vi "identColor.vi"(7 "Parâmetros Ini":T2={"Gyro Port"=0, "Sensor - Left"=3, "Sensor - Right"=2, "     Color \nSensor Port"=1, "Kp Front"=0.5, "Motor speed"=-15, "Distance to street"=0.0, "Motor speed turns"=16, "Kp Curvas"=0.0} {"Kp Front" format="%.3f"; "Color \nSensor Port" items=["Port 1", "Port 2", "Port 3", "Port 4"]; "Sensor - Right" items=["Port 1", "Port 2", "Port 3", "Port 4"]; "Sensor - Left" items=["Port 1", "Port 2", "Port 3", "Port 4"]; "Gyro Port" items=["Port 1", "Port 2", "Port 3", "Port 4"]}, 11 "NXT/EV3":T1) -> (1 "Collor":T4)   [LabVIEW 2016]
uses:
  <vilib>/NXT/Subs/LVHSConnector.ctl
  <vilib>/NXT/LegoClasses/BrickReference/BrickReference.lvclass
  <vilib>/NXT/Subs/ColorSensorColors.ctl
  parametros.ctl
  <vilib>/NXT/Block Support/NXT_InputPort.ctl
panel:
  out "NXT/EV3 2":T1
  out "Detected Color":T4
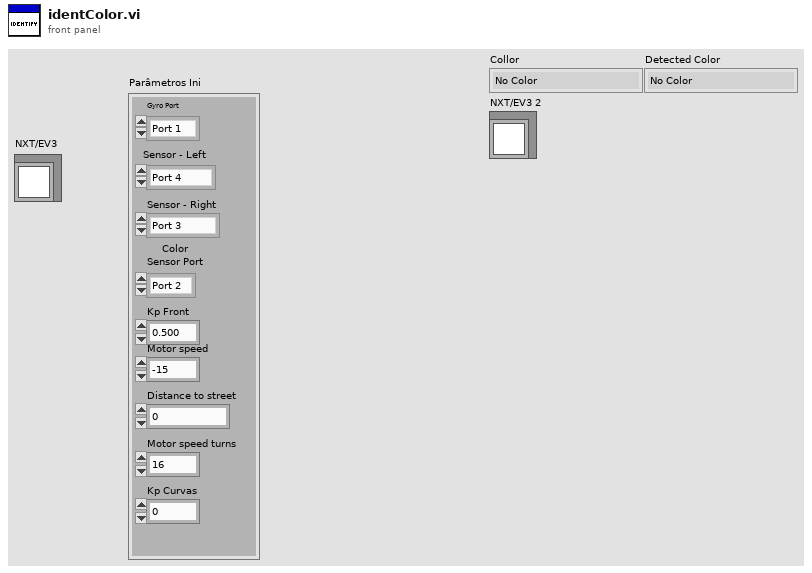
[diagram p1: front panel]
types:
  T1 = typedef "LVHSConnector.ctl" = refnum<class "BrickReference.lvclass">
  T2 = typedef "parametros.ctl" = cluster{"Gyro Port":T3, "Sensor - Left":T3, "Sensor - Right":T3, "     Color \nSensor Port":T3, "Kp Front":dbl, "Motor speed":i32, "Distance to street":dbl, "Motor speed turns":i32, "Kp Curvas":dbl}
  T3 = typedef "NXT_InputPort.ctl" = u32
  T4 = typedef "ColorSensorColors.ctl" = enum16{"No Color", "Black", "Blue", "Green", "Yellow", "Red", "White", "Brown"}
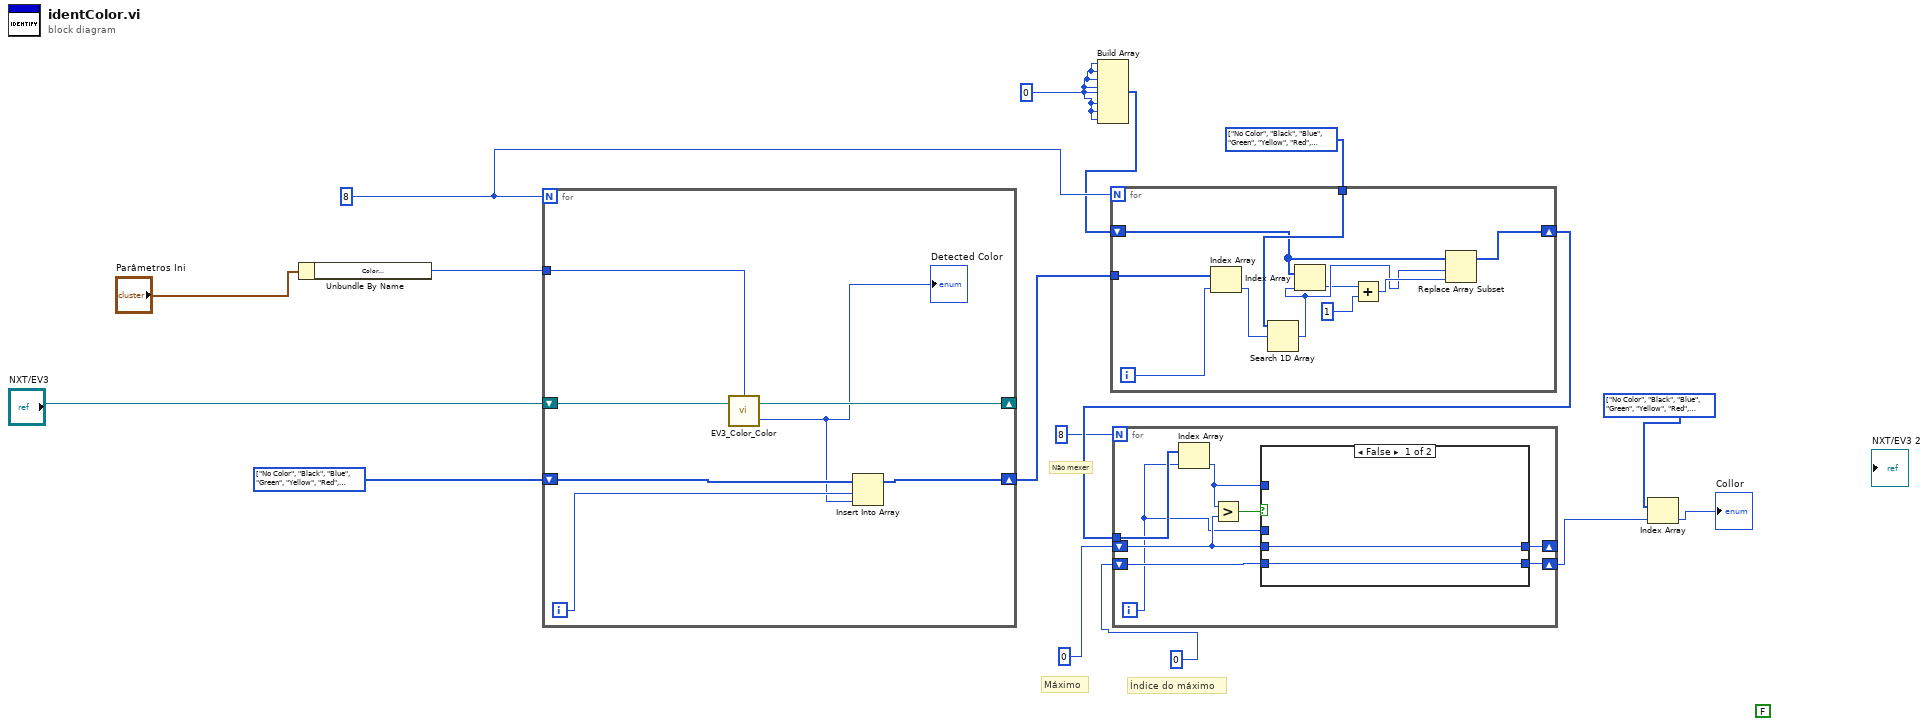
[diagram p0: block diagram]
diagram:
  (unwired) FALSE ("stop")
  w4 = 0
  w5 = T4[] [enum."No Color", enum."Black", enum."Blue", enum."Green", enum."Yellow", enum."Red", enum."White", enum."Brown"] items=["No Color", "Black", "Blue", "Green", "Yellow", "Red", "White", "Brown"]
  w6 = T4[] [enum."No Color", enum."Black", enum."Blue", enum."Green", enum."Yellow", enum."Red", enum."White", enum."Brown"] items=["No Color", "Black", "Blue", "Green", "Yellow", "Red", "White", "Brown"]
  w13 = 8
  w15 = T4[] [enum."No Color", enum."Black", enum."Blue", enum."Green", enum."Yellow", enum."Red", enum."White", enum."Blue"] items=["No Color", "Black", "Blue", "Green", "Yellow", "Red", "White", "Brown"]
  # "Não mexer"
  # "Índice do máximo"
  # "Máximo"
  n1 = Unbundle By Name("Parâmetros Ini") -> ("Color \nSensor Port"=w1:T3)
  n2 = for {
    N: w13 -> [_]
    shift-right: [w19] -> _
    shift-left: "NXT/EV3" -> [w20]
    shift-right: [w21] -> w14
    shift-left: w5 -> [w22]
    tunnel: w1 -> [w18]
    i -> [w23]
    n3 = call <vilib>:"EV3_Color_Color.vi"("NXT/EV3"=w20, "Port (Port 1)"=w18) -> ("Detected Color"=w17:T4, "NXT/EV3"=w19:T1)  [unwired: 1 in]
    "Detected Color" <- w17
    n4 = Insert Into Array(array=w22, index=w23, new element=w17) -> (w21:T4[])
  }
  n5 = Build Array(w4, w4, w4, w4, w4, w4, w4, w4) -> (w3:i32[])
  n6 = for {
    N: w13 -> [_]
    tunnel: w14 -> [w32]
    shift-right: [w29] -> w12
    shift-left: w3 -> [w25]
    tunnel: w6 -> [w27]
    i -> [w33]
    n7 = Index Array(array=w32, index=w33) -> (element=w28:T4)
    n8 = Search 1D Array(1D array=w27, element=w28) -> (index of element=w26:i32)  [unwired: 1 in]
    n9 = Index Array(array=w25, index=w26) -> (element=w24:i32)
    n10 = Add(x=w24, y=1) -> (x+y=w30:i32)
    n11 = Replace Array Subset(array=w25, new element=w30, index=w26) -> (w29:i32[])
  }
  n12 = for {
    N: 8 -> [_]
    tunnel: w12 -> [w41]
    shift-right: [w39] -> _
    shift-left: 0 -> [w36]
    shift-right: [w37] -> w8
    shift-left: 0 -> [w35]
    i -> [w34]
    n13 = Index Array(array=w41, index=w34) -> (element=w38:i32)
    n14 = Greater?(x=w38, y=w36) -> (0:w40:bool)
    n15 = case shown="False" w40 {
      tunnel: w36 -> [w43 _]
      tunnel: [w43 w45] -> w39
      tunnel: w38 -> [_ w45]
      tunnel: [w42 w44] -> w37
      tunnel: w35 -> [w42 _]
      tunnel: w34 -> [_ w44]
      frame False {
      }
      frame True {
      }
    }
  }
  n16 = Index Array(array=w15, index=w8) -> (element=→"Collor":T4)
